vi "CMN_toLogical.vi"(9 "command":string) -> ()   [LabVIEW 2016]
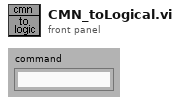
[diagram p1: front panel]
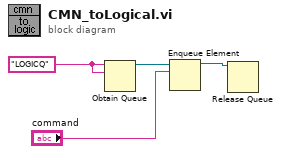
[diagram p0: block diagram]
diagram:
  w4 = "LOGICQ" ("name (unnamed)")
  n1 = Obtain Queue(name (unnamed)=w4, element data type=w4) -> (queue out=w3:refnum<queue>)  [unwired: 3 in, 2 out]
  n2 = Enqueue Element(queue=w3, element="command") -> (queue out=w1:refnum<queue>)  [unwired: 1 in, 3 out]
  n3 = Release Queue(queue=w1) -> ()  [unwired: 1 in, 4 out]
